vi "DIM_DIO.ProcEvents.vi"(0 "i ref in":refnum<vi>, 5 "error in (no error)":errorcluster) -> (14 "i ref out":refnum<vi>, 19 "error out":errorcluster)   [LabVIEW 2014, in "DIM_DIO.lvlib"]
doc: "This method is used to define the events the object will listen to. Add your own events here."
uses:
  DIM_DIO.lvlib
  CSCore/CAEObj/CAEObj.event definition.ctl
  CSCore/BaseProcess/BaseProcess.event definition.ctl
  CSCore/BaseProcess/BaseProcess.descriptor string definition.ctl
  CSCore/BaseProcess/BaseProcess.lvlib
  CSCore/CAEObj/CAEObj.lvlib
panel:
  in  "event definition type":T1
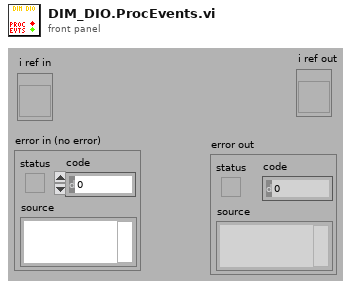
[diagram p1: front panel]
types:
  T1 = typedef "CAEObj.lvlib/CAEObj.event definition.ctl" = cluster{"URL":string, "enable":bool, "ignoreResID":bool}
  T2 = typedef "BaseProcess.lvlib/BaseProcess.event definition.ctl" = cluster{"CAEEvtDef":T1, "Data Descriptor":T3}
  T3 = typedef "BaseProcess.lvlib/BaseProcess.descriptor string definition.ctl" = string
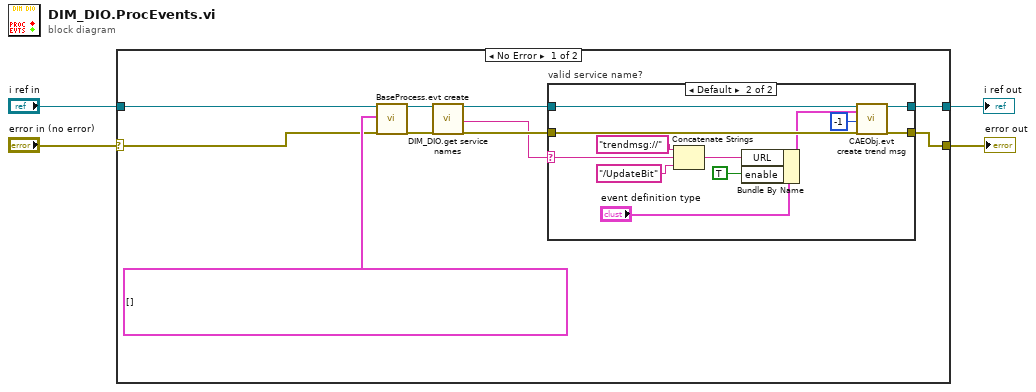
[diagram p0: block diagram]
diagram:
  n1 = case shown="No Error" "error in (no error)" {
    selector: "error in (no error)" -> [w12 w29]
    tunnel: "i ref in" -> [w14 w30]
    tunnel: [w8 w30] -> w3
    tunnel: [w6 w29] -> w2
    frame No Error {
      n2 = call "BaseProcess.evt create.vi"("i ref in"=w14, "newEvents"=T2[] [] ("new events"), "error in (no error)"=w12) -> ("i ref out"=w11:refnum<vi>, "error out"=w10:errorcluster)  [unwired: 13 in, 2 out]
      n3 = call "DIM_DIO.get service names.vi"("i ref in"=w11, "error in (no error)"=w10) -> ("i ref out"=w9:refnum<vi>, "readService"=w5:string, "error out"=w7:errorcluster)  [unwired: 14 in, 1 out]
      n4 = case "valid service name?" shown="Default" w5 {
        selector: w5 -> [_ w17]
        tunnel: w9 -> [w16 w25]
        tunnel: [w16 w24] -> w8
        tunnel: w7 -> [w15 w23]
        tunnel: [w15 w22] -> w6
        frame "N/A" {
        }
        frame Default {
          n5 = Concatenate Strings("trendmsg://" ("string"), w17, "/UpdateBit" ("string")) -> (w21:string)
          n6 = Bundle By Name(cluster="event definition type", "URL"=w21, "enable"=TRUE) -> (w18:T1)
          n7 = call "CAEObj.evt create trend msg.vi"("i ref in"=w25, "event definition"=w18, "ms timeout (10000)"=-1 ("ms timeout (100)"), "error in (no error)"=w23) -> ("i ref out"=w24:refnum<vi>, "error out"=w22:errorcluster)  [unwired: 12 in, 2 out]
        }
      }
    }
    frame Error {
    }
  }
  "i ref out" <- w3
  "error out" <- w2
